vi "VWflipperArray.vi"(7 "Theta Degree":dbl[](array[numeric]), 8 "Probe w m/s":dbl[](array[numeric]), 9 "Probe v m/s":dbl[](array[numeric]), 10 "Probe u  m/s":dbl[](array[numeric]), 11 "VMagn m/s":dbl[](array[numeric])) -> (3 "VmagUVWCone":dbl[][](array[numeric]))   [LabVIEW 2013]
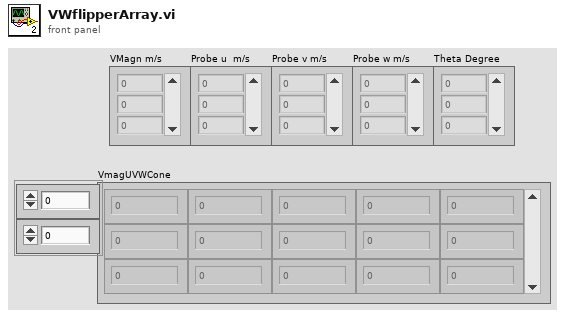
[diagram p1: front panel]
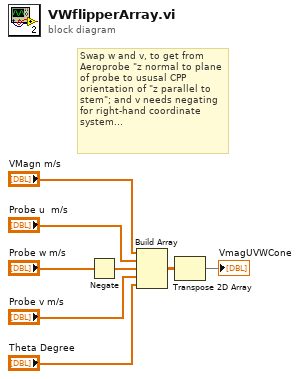
[diagram p0: block diagram]
diagram:
  # "Swap w and v, to get from Aeroprobe \"z normal to plane of probe to ususal CPP orientation of \"z parallel to stem\"; and v needs negating for right-hand coordinate system..."
  n1 = Negate(x="Probe w m/s") -> (-x=w5:dbl[])
  n2 = Build Array("VMagn m/s", "Probe u  m/s", w5, "Probe v m/s", "Theta Degree") -> (w2:dbl[][])
  n3 = Transpose 2D Array(2D array=w2) -> (transposed array=→"VmagUVWCone":dbl[][])
